vi "Do That Thang.vi"(7 "Test Executive Ref out":refnum<data-value>, 10 "error in (no error)":errorcluster, 11 "Executioner in":refnum<class "Executioner.lvclass">) -> (2 "error out":errorcluster)   [LabVIEW 2017, in "Nested Conditional in While Loop Example.lvlib" / "iTest Step.lvclass"]
uses:
  <vilib>/gpm_packages/@cs/test-executive/Source/Sandbox/Nested Conditional in While Loop Example/iTest Step/iTest Step.lvclass
  <vilib>/gpm_packages/@cs/test-executive/Source/Test Executive/Executioner/Executioner.lvclass
  <vilib>/gpm_packages/@cs/test-executive/Source/Test Executive/ITestExecutive/ITest Executive.lvclass
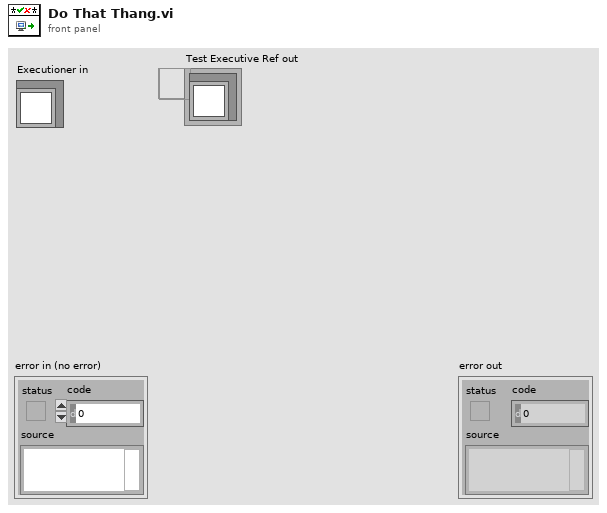
[diagram p1: front panel]
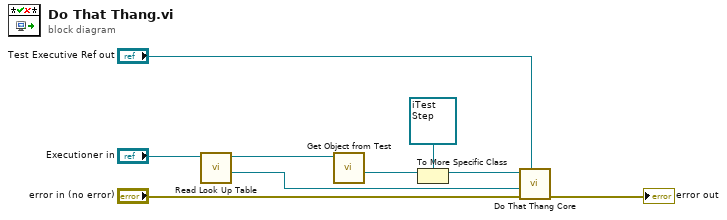
[diagram p0: block diagram]
diagram:
  n1 = call <vilib>:"Read Look Up Table.vi"("Executioner in"="Executioner in") -> ("Attributes Ref"=w1:refnum<data-value>, "Executioner out"=w9:refnum<class "Executioner.lvclass">)  [unwired: 9 in]
  n2 = call <vilib>:"Get Object from Test.vi"("Executioner in"=w9) -> ("Test"=w7:refnum<class>)  [unwired: 9 in, 1 out]
  n3 = To More Specific Class(target class=refnum<class "iTest Step.lvclass"> refnum ("iTest Step in"), reference=w7) -> (specific class reference=w5:refnum<class "iTest Step.lvclass">)  [unwired: 1 in, 1 out]
  n4 = call-dynamic "Do That Thang Core.vi"("Test Executive Ref out"="Test Executive Ref out", "error in (no error)"="error in (no error)", "Attributes Ref"=w1, "iTest Step in"=w5) -> ("error out"=→"error out":errorcluster)  [unwired: 7 in]
